vi "Test DBModule API.vi"() -> ()   [LabVIEW 2022 SP3]
doc: "DBModule API Tester.\n\n<b>Note:</b> This VI was modified by the <b>Validate DQMH Module</b> tool to add the 'Show Main VI Diagram on Init' functionality included in DQMH 6.1.\n\n<b>Note:</b> This VI was modified by the <b>Validate DQMH Module</b> tool to upgrade its Error Reported event frame to use an improved mechanism for displaying error information.\n\n____\nHAMPEL SOFTWARE ENGINEERING v2.6.0 (2023-12-19 10:54)"
uses:
  Libraries/hse-libraries/Source/hse-dqmh/Controls/Module Display Scenarios.ctl
  <vilib>/Utility/error.llb/DialogType.ctl
  <vilib>/Hampel Software Engineering/HSE Logger/LogRecord/LogRecord.lvclass/LogRecord.ctl
  DBModule.lvlib
  Libraries/hse-libraries/Source/hse-dqmh/hse-dqmh.lvlib
  <vilib>/Hampel Software Engineering/HSE Logger/LogRecord/LogRecord.lvclass
  <vilib>/Hampel Software Engineering/HSE Logger/hse-logger.lvlib
panel:
  in  "Show Main VI Diagram on Init (F)":bool
  in  "Scenario":T1
  in  "Request UI Display":bool
  in  "Prepare":bool
  in  "Configure":bool
  in  "Show Block Diagram":bool
  in  "Stop Module":bool
  in  "Start Module":bool
  in  "Hide Module Panel":bool
  in  "Show Module Panel":bool
  out "Status":string
  out "Module Running?":bool
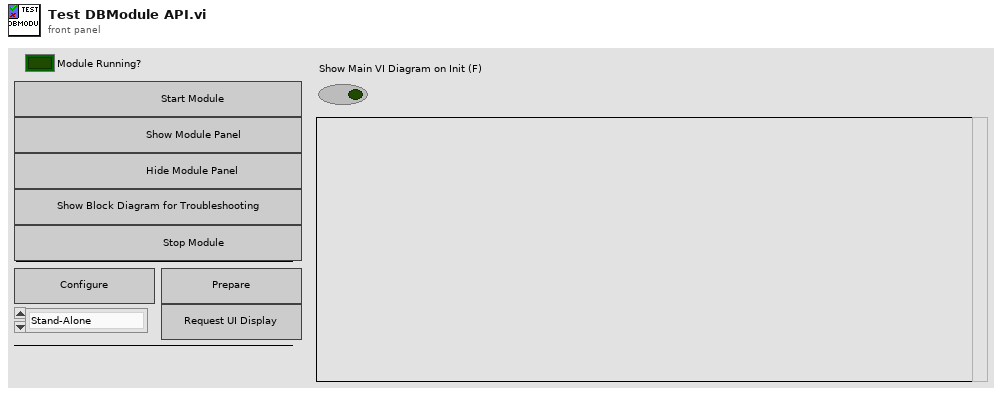
[diagram p1: front panel]
types:
  T1 = typedef "hse-dqmh.lvlib/Module Display Scenarios.ctl" = enum16{"Stand-Alone", "Managed"}
  T2 = typedef "DBModule.lvlib/Broadcast Events--cluster.ctl" = cluster{"Module Did Init":refnum<user-event>, "Status Updated":refnum<user-event>, "Error Reported":refnum<user-event>, "Module Did Stop":refnum<user-event>, "Update Module Execution Status":refnum<user-event>, "System Message":refnum<user-event>}
  T3 = typedef "DialogType.ctl" = u16
  T4 = typedef "hse-dqmh.lvlib/System Message Source.ctl" = enum16{"module", "application", "network"}
  T5 = typedef "hse-logger.lvlib/LogLevel.ctl" = enum16{"DEBUG", "INFO", "WARNING", "ERROR", "CRITICAL"}
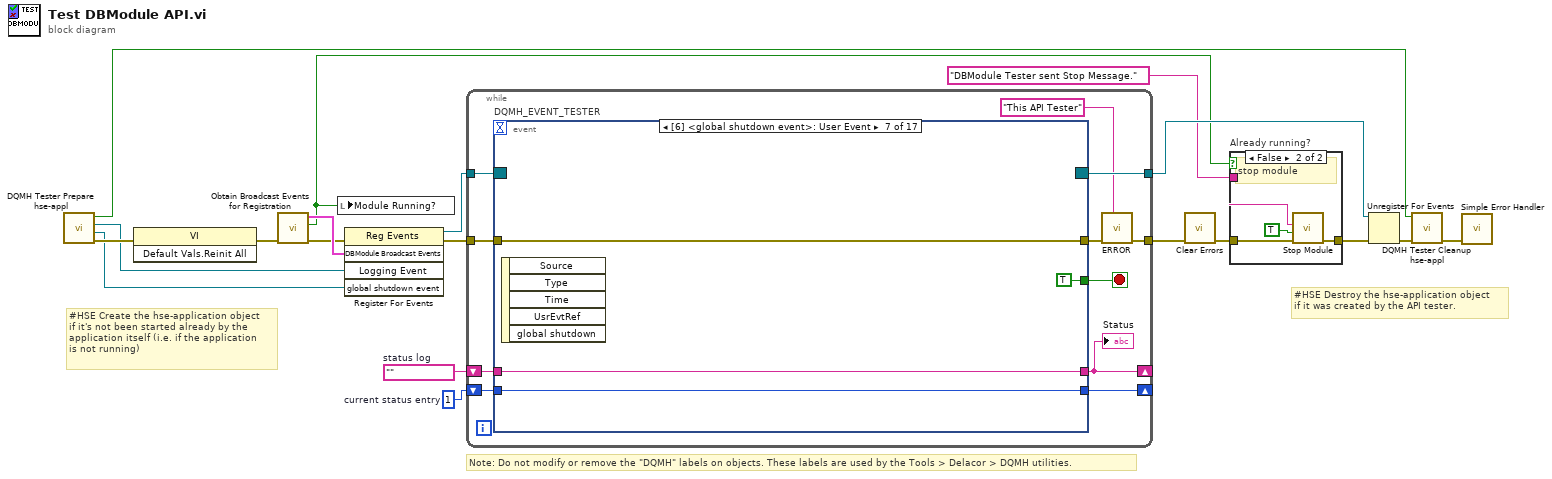
[diagram p0: block diagram]
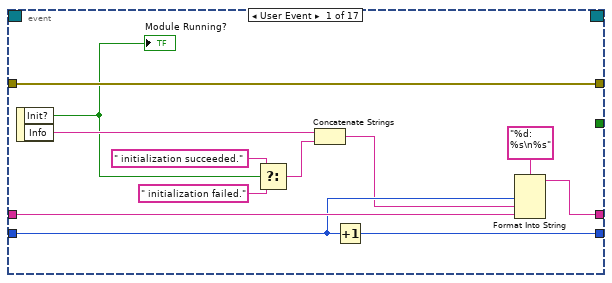
[diagram p3: hidden frame]
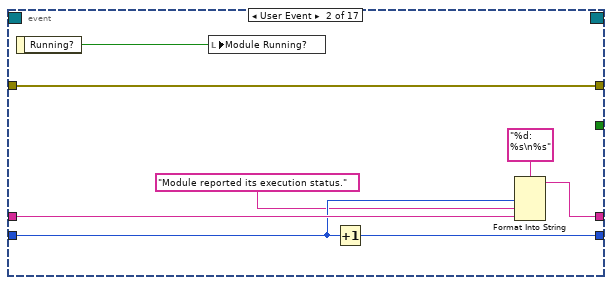
[diagram p4: hidden frame]
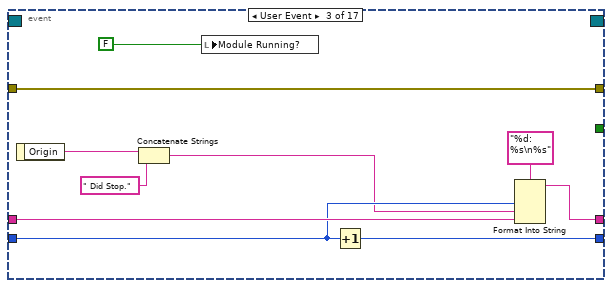
[diagram p5: hidden frame]
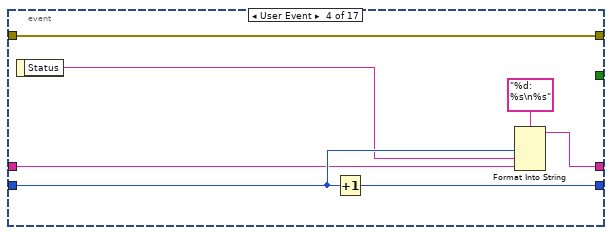
[diagram p6: hidden frame]
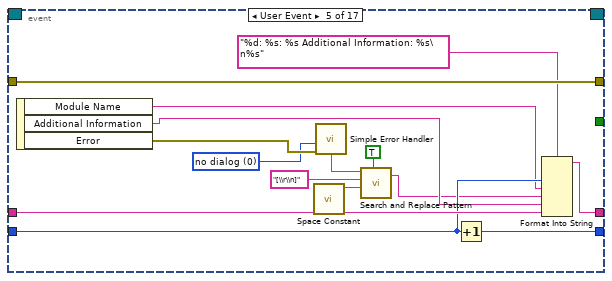
[diagram p7: hidden frame]
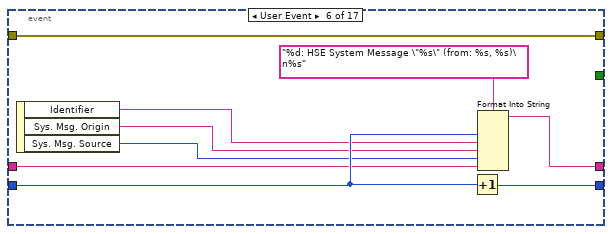
[diagram p8: hidden frame]
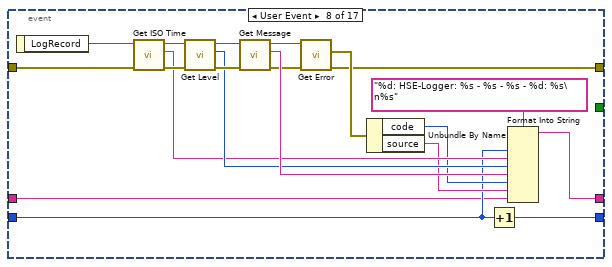
[diagram p9: hidden frame]
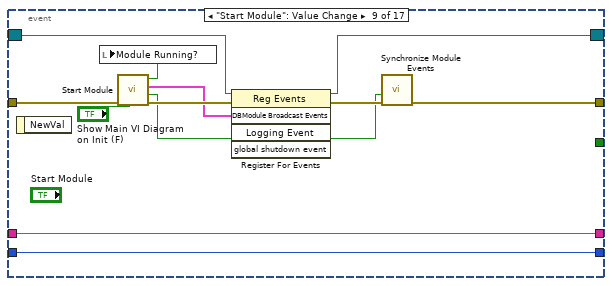
[diagram p10: hidden frame]
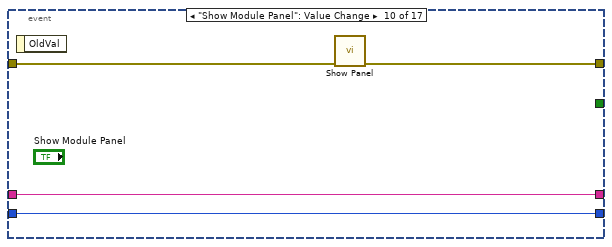
[diagram p11: hidden frame]
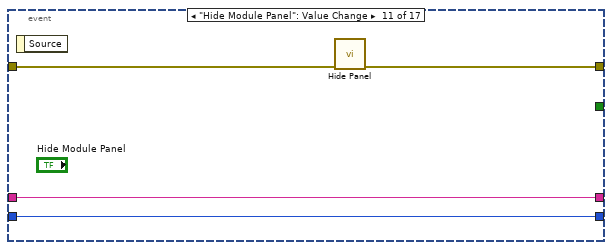
[diagram p12: hidden frame]
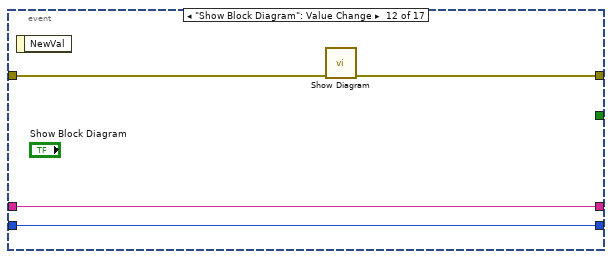
[diagram p13: hidden frame]
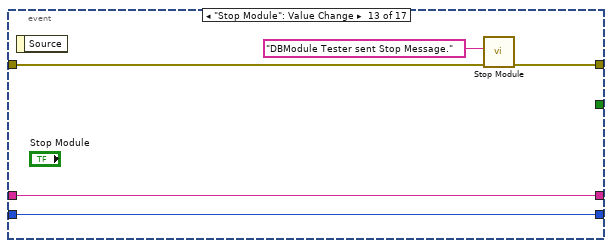
[diagram p14: hidden frame]
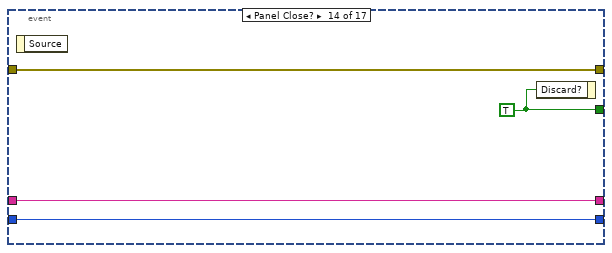
[diagram p15: hidden frame]
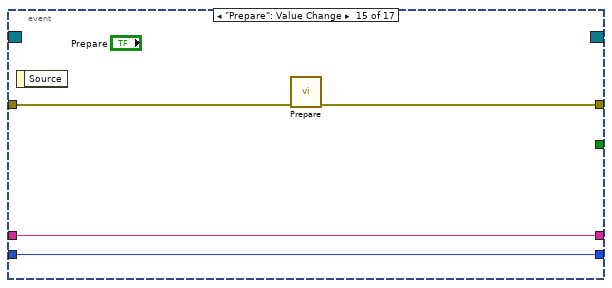
[diagram p16: hidden frame]
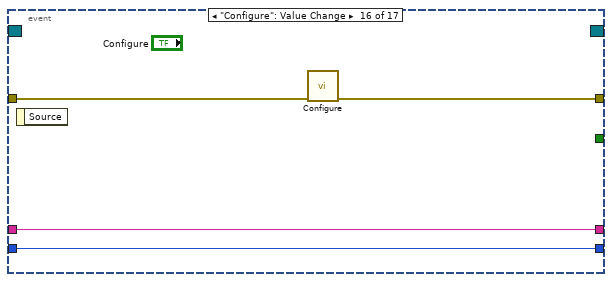
[diagram p17: hidden frame]
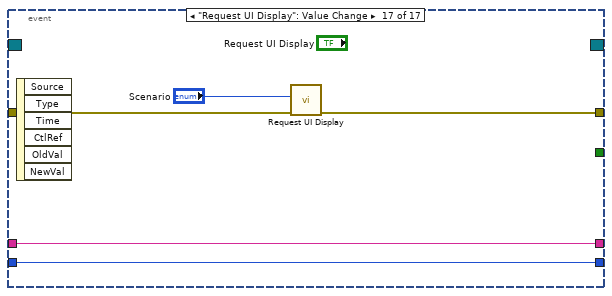
[diagram p18: hidden frame]
diagram:
  w17 = 1  # current status entry
  w18 = ""  # status log
  # "#HSE Destroy the hse-application object\nif it was created by the API tester."
  # "#HSE Create the hse-application object\nif it's not been started already by the \napplication itself (i.e. if the application\nis not running)"
  # "Note: Do not modify or remove the \"DQMH\" labels on objects. These labels are used by the Tools > Delacor > DQMH utilities."
  n1 = call "DQMH Tester Prepare hse-appl.vi"() -> ("error out"=w7:errorcluster, "global shutdown event"=w1:refnum<user-event>, "Logging Event"=w6:refnum<user-event>, "Started?"=w4:bool)  [unwired: 8 in]
  n2 = invoke class="VI" method="Default Vals.Reinit All"(error in=w7) -> (error out=w9:errorcluster)  [unwired: 2 in, 2 out]
  n3 = call "Obtain Broadcast Events for Registration.vi"("error in (no error)"=w9) -> ("error out"=w8:errorcluster, "Already running?"=w10:bool, "DBModule Broadcast Events"=w15:T2)  [unwired: 8 in]
  n4 = local write "Module Running?"(w10) -> ()
  n5 = register-events(error in=w8, w15, w6, w1) -> (reference out=w14:refnum<event-registration>, error out=w16:errorcluster)  [unwired: 1 in]
  n6 = while {
    tunnel: w14 -> [w30]
    tunnel: [w21] -> w11
    shift-right: [w26] -> _
    shift-left: w18 -> [w28]
    shift-right: [w27] -> _
    shift-left: w17 -> [w29]
    tunnel: w16 -> [w25]
    tunnel: [w24] -> w13
    stop <- w23 stop-if-true
    n7 = event "DQMH_EVENT_TESTER" shown="[6] <global shutdown event>: User Event" {
      selector: w30 -> [_ _ _ _ _ _ _ _ w121 _ _ _ _ _ _ _ _]
      dyn-events: [_ _ _ _ _ _ _ _ w120 _ _ _ _ _ _ _ _] -> w24
      timeout: _ -> [_ _ _ _ _ _ _ _ _ _ _ _ _ _ _ _ _]
      tunnel: [_ _ _ _ _ _ TRUE ("Discard?") _ _ _ _ _ _ w148 _ _ _] -> w23
      tunnel: [w42 w44 w51 w61 w82 w91 w95 w96 w117 w131 w135 w136 w142 w145 w149 w153 w158] -> w22
      tunnel: w29 -> [w39 w48 w58 w64 w79 w87 w93 w102 w124 w129 w133 w137 w143 w146 w150 w155 w159]
      tunnel: w28 -> [w40 w49 w59 w63 w81 w86 w94 w101 w125 w130 w134 w138 w144 w147 w151 w156 w160]
      tunnel: [w37 w46 w56 w65 w80 w89 w94 w99 w125 w130 w134 w138 w144 w147 w151 w156 w160] -> w26
      tunnel: [w38 w47 w57 w67 w78 w88 w93 w100 w124 w129 w133 w137 w143 w146 w150 w155 w159] -> w27
      tunnel: w25 -> [w42 w44 w51 w61 w82 w91 w95 w97 w119 w128 w132 w139 w140 w145 w152 w154 w161]
      event User Event {
        n8 = event-data() -> ("Init?"=w34:bool, "Info"=w36:string)  [unwired: 1 in]
        "Module Running?" <- w34
        n9 = Select(t=" initialization succeeded.", s=w34, f=" initialization failed.") -> (s? t:f=w31:string)
        n10 = Concatenate Strings(w36, w31) -> (w35:string)
        n11 = Increment(x=w39) -> (x+1=w38:i32)
        n12 = Format Into String(format string="%d: %s\n%s", w39, w35, w40) -> (resulting string=w37:string)  [unwired: 2 in, 1 out]
      }
      event User Event {
        n13 = event-data() -> ("Running?"=w43:bool)  [unwired: 1 in]
        n14 = local write "Module Running?"(w43) -> ()
        n15 = Increment(x=w48) -> (x+1=w47:i32)
        n16 = Format Into String(format string="%d: %s\n%s", w48, "Module reported its execution status.", w49) -> (resulting string=w46:string)  [unwired: 2 in, 1 out]
      }
      event User Event {
        n17 = event-data() -> ("Origin"=w55:string)  [unwired: 1 in]
        n18 = Concatenate Strings(w55, " Did Stop.") -> (w54:string)
        n19 = local write "Module Running?"(FALSE ("Module Did Init?")) -> ()
        n20 = Increment(x=w58) -> (x+1=w57:i32)
        n21 = Format Into String(format string="%d: %s\n%s", w58, w54, w59) -> (resulting string=w56:string)  [unwired: 2 in, 1 out]
      }
      event User Event {
        n22 = event-data() -> ("Status"=w62:string)  [unwired: 1 in]
        n23 = Increment(x=w64) -> (x+1=w67:i32)
        n24 = Format Into String(format string="%d: %s\n%s", w64, w62, w63) -> (resulting string=w65:string)  [unwired: 2 in, 1 out]
      }
      event User Event {
        w74 = T3 0 items=["no dialog", "OK message", "continue or stop message", "OK message + warnings", "continue/stop + warnings"] ("type of dialog (OK msg:1)")
        n25 = event-data() -> ("Module Name"=w75:string, "Additional Information"=w76:string, "Error"=w77:errorcluster)  [unwired: 1 in]
        n26 = call <vilib>:"Space Constant.vi"() -> ("String"=w70:string)
        n27 = call <vilib>:"Simple Error Handler.vi"("type of dialog (OK msg:1)"=w74, "error in (no error)"=w77) -> ("message"=w73:string)  [unwired: 3 in, 4 out]
        n28 = call <vilib>:"Search and Replace Pattern.vi"("string"=w73, "regular expression (\"\")"="[\\r\\n]" ("regular expression (\"\")"), "replace string (\"\")"=w70, "replace all? (F)"=TRUE ("replace all CR/LF with spaces")) -> ("result string"=w72:string)  [unwired: 1 in, 1 out]
        n29 = Increment(x=w79) -> (x+1=w78:i32)
        n30 = Format Into String(format string="%d: %s: %s Additional Information: %s\n%s", w79, w75, w72, w76, w81) -> (resulting string=w80:string)  [unwired: 2 in, 1 out]
      }
      event User Event {
        n31 = event-data() -> ("Identifier"=w85:string, "Sys. Msg. Origin"=w84:string, "Sys. Msg. Source"=w83:T4)  [unwired: 1 in]
        n32 = Increment(x=w87) -> (x+1=w88:i32)
        n33 = Format Into String(format string="%d: HSE System Message \"%s\" (from: %s, %s)\n%s", w87, w85, w84, w83, w86) -> (resulting string=w89:string)  [unwired: 2 in, 1 out]
      }
      event User Event {
        n34 = event-data() -> ()  [unwired: 1 in, 5 out]
      }
      event User Event {
        n35 = event-data() -> ("LogRecord"=w98:refnum<class "LogRecord.lvclass">)  [unwired: 1 in]
        n36 = call <vilib>:"Get ISO Time.vi"("error in"=w97, "LogRecord in"=w98) -> ("error out"=w107:errorcluster, "ISO Time"=w106:string, "LogRecord out"=w109:refnum<class "LogRecord.lvclass">)  [unwired: 7 in]
        n37 = call <vilib>:"Get Level.vi"("error in"=w107, "LogRecord in"=w109) -> ("error out"=w110:errorcluster, "Level"=w108:T5, "LogRecord out"=w111:refnum<class "LogRecord.lvclass">)  [unwired: 7 in]
        n38 = call <vilib>:"Get Message.vi"("error in"=w110, "LogRecord in"=w111) -> ("error out"=w112:errorcluster, "Message"=w115:string, "LogRecord out"=w113:refnum<class "LogRecord.lvclass">)  [unwired: 7 in]
        n39 = call <vilib>:"Get Error.vi"("error in"=w112, "LogRecord in"=w113) -> ("error out"=w96:errorcluster, "Error"=w114:errorcluster)  [unwired: 7 in, 1 out]
        n40 = Unbundle By Name(w114) -> ("code"=w104:i32, "source"=w105:string)
        n41 = Increment(x=w102) -> (x+1=w100:i32)
        n42 = Format Into String(format string="%d: HSE-Logger: %s - %s - %s - %d: %s\n%s", w102, w106, w108, w115, w104, w105, w101) -> (resulting string=w99:string)  [unwired: 2 in, 1 out]
      }
      event "Start Module": Value Change {
        n43 = event-data() -> ()  [unwired: 1 in, 1 out]
        n44 = call "Start Module.vi"("Show Main VI Diagram on Init (F)"="Show Main VI Diagram on Init (F)", "error in (no error)"=w119) -> ("error out"=w126:errorcluster, "Wait for Event Sync?"=w123:bool, "DBModule Broadcast Events"=w122:T2, "Module Was Already Running?"=w118:bool)  [unwired: 6 in]
        n45 = local write "Module Running?"(w118) -> ()
        n46 = register-events(reference=w121, error in=w126, w122) -> (reference out=w120:refnum<event-registration>, error out=w127:errorcluster)  [unwired: 2 in]
        n47 = call "Synchronize Module Events.vi"("error in (no error)"=w127, "Wait for Event Sync?"=w123) -> ("error out"=w117:errorcluster)  [unwired: 9 in]
      }
      event "Show Module Panel": Value Change {
        n48 = event-data() -> ()  [unwired: 1 in, 1 out]
        n49 = call "Show Panel.vi"("error in (no error)"=w128) -> ("error out"=w131:errorcluster)  [unwired: 10 in]
      }
      event "Hide Module Panel": Value Change {
        n50 = event-data() -> ()  [unwired: 1 in, 1 out]
        n51 = call "Hide Panel.vi"("error in (no error)"=w132) -> ("error out"=w135:errorcluster)  [unwired: 10 in]
      }
      event "Show Block Diagram": Value Change {
        n52 = event-data() -> ()  [unwired: 1 in, 1 out]
        n53 = call "Show Diagram.vi"("error in (no error)"=w139) -> ("error out"=w136:errorcluster)  [unwired: 10 in]
      }
      event "Stop Module": Value Change {
        n54 = event-data() -> ()  [unwired: 1 in, 1 out]
        n55 = call "Stop Module.vi"("error in (no error)"=w140, "Origin"="DBModule Tester sent Stop Message.") -> ("error out"=w142:errorcluster)  [unwired: 9 in]
      }
      event Panel Close? {
        w148 = TRUE ("Discard?")
        n56 = event-data() -> ()  [unwired: 1 in, 1 out]
        n57 = event-data("Discard?"=w148) -> ()  [unwired: 1 in, 1 out]
      }
      event "Prepare": Value Change {
        n58 = event-data() -> ()  [unwired: 1 in, 1 out]
        n59 = call "Prepare.vi"("error in (no error)"=w152) -> ("error out"=w149:errorcluster)  [unwired: 10 in]
      }
      event "Configure": Value Change {
        n60 = event-data() -> ()  [unwired: 1 in, 1 out]
        n61 = call "Configure.vi"("error in (no error)"=w154) -> ("error out"=w153:errorcluster)  [unwired: 10 in]
      }
      event "Request UI Display": Value Change {
        n62 = event-data() -> ()  [unwired: 1 in, 6 out]
        n63 = call "Request UI Display.vi"("error in (no error)"=w161, "Scenario"="Scenario") -> ("error out"=w158:errorcluster)  [unwired: 8 in, 1 out]
      }
    }
    "Status" <- w26
    n64 = call <vilib>:"ERROR.vi"("Message"="This API Tester" ("Origin"), "error in"=w22) -> ("error out"=w21:errorcluster)  [unwired: 9 in]
  }
  n65 = call <vilib>:"Clear Errors.vi"("error in (no error)"=w11) -> ("error out"=w12:errorcluster)  [unwired: 5 in, 1 out]
  n66 = case "Already running?" shown="False" w10 {
    tunnel: [w162 w166] -> w19
    tunnel: w12 -> [w162 w164]
    tunnel: "DBModule Tester sent Stop Message." ("Origin") -> [_ w163]
    frame True {
      # "don't stop"
    }
    frame False {
      # "stop module"
      n67 = call "Stop Module.vi"("error in (no error)"=w164, "Wait for Module to Stop? (F)"=TRUE ("Wait for Module to stop?"), "Origin"=w163) -> ("error out"=w166:errorcluster)  [unwired: 8 in]
    }
  }
  n68 = Unregister For Events(event registration refnum=w13, error in=w19) -> (error out=w5:errorcluster)
  n69 = call "DQMH Tester Cleanup hse-appl.vi"("error in"=w5, "Stop?"=w4) -> ("error out"=w2:errorcluster)  [unwired: 9 in]
  n70 = call <vilib>:"Simple Error Handler.vi"("error in (no error)"=w2) -> ()  [unwired: 4 in, 5 out]
